vi "HDPE Export Coordinates.vi"(8 "error in (no error)":errorcluster, 9 "Image Index":i32, 10 "Image Path Array":path[](array[path]), 11 "Rectangle Coordinates":dbl[][](array[numeric])) -> (0 "error out":errorcluster)   [LabVIEW 2019]
uses:
  <vilib>/Utility/file.llb/Write Delimited Spreadsheet (DBL).vi
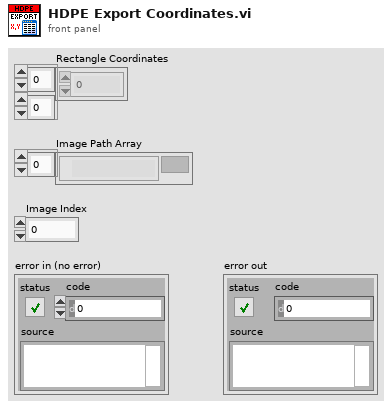
[diagram p1: front panel]
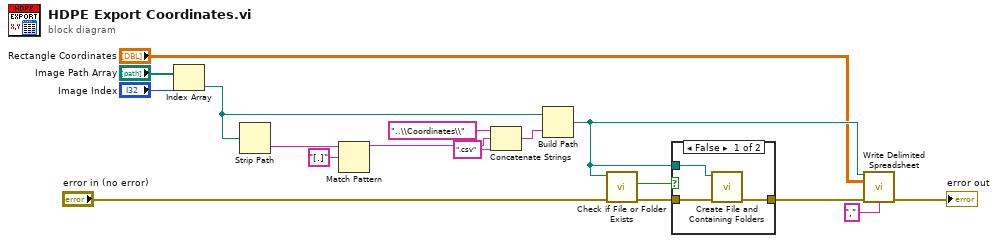
[diagram p0: block diagram]
diagram:
  n1 = Index Array(array="Image Path Array", index="Image Index") -> (element=w12:path)
  n2 = Strip Path(path=w12) -> (name=w3:string)  [unwired: 1 out]
  n3 = Match Pattern(string=w3, regular expression="[.]") -> (before substring=w7:string)  [unwired: 1 in, 3 out]
  n4 = Concatenate Strings("..\\Coordinates\\" ("name or relative path"), w7, ".csv" ("string")) -> (w6:string)
  n5 = Build Path(base path=w12, name or relative path=w6) -> (appended path=w17:path)
  n6 = call <vilib>:"Check if File or Folder Exists.vi"("error in (no error)"="error in (no error)", "path"=w17) -> ("error out"=w15:errorcluster, "file or folder exists?"=w16:bool)  [unwired: 7 in, 1 out]
  n7 = case shown="False" w16 {
    tunnel: [w20 w21] -> w9
    tunnel: w15 -> [w19 w21]
    tunnel: w17 -> [w18 _]
    frame False {
      n8 = call <vilib>:"Create File and Containing Folders.vi"("error in (no error)"=w19, "file path"=w18) -> ("error out"=w20:errorcluster)  [unwired: 8 in, 1 out]
    }
    frame True {
    }
  }
  n9 = call-poly <vilib>:"Write Delimited Spreadsheet.vi"("file path (dialog if empty)"=w17, "2D data"="Rectangle Coordinates", "error in (no error)"=w9, "delimiter (\\t)"="," ("delimiter (\\t)")) -> ("error out"=→"error out":errorcluster)  [unwired: 10 in, 1 out]
